vi "RunInference.vi"(4 "Output Index":i32, 6 "Input Index":i32, 7 "DLL path":path, 8 "error in (no error)":errorcluster, 9 "Output Buffer":sgl[](array[numeric]), 10 "Input Buffer":sgl[](array[numeric]), 11 "session id in":i32) -> (0 "error out":errorcluster, 2 "outputBuffer":sgl[](array[numeric]), 3 "session id out":i32)   [LabVIEW 2017, in "ONNX Class Library.lvlib"]
doc: "/**\n * @brief Выполнить инференс (предсказание) модели\n * \n * Основная функция для получения предсказания от модели. Принимает входные данные,\n * передаёт их в нейросеть и записывает результат в выходной буфер.\n * \n * @param sessionId [IN] ID сессии\n * @param inputIndex [IN] Индекс входа (обычно 0 для моделей с одним входом)\n * @param inputBuffer [IN] Массив входных данных (тип должен соответствовать GetInputType)\n * @param inputSize [IN] Количество элементов во входном массиве\n * @param outputIndex [IN] Индекс выхода (обычно 0 для моделей с одним выходом)\n * @param outputBuffer [OUT] Массив для записи результатов (должен быть выделен в LabVIEW)\n * @param outputSize [IN] Размер выходного буфера в элементах\n * \n * @return int32: 0 при успешном выполнении инференса\n * @return int32: -1 при ошибке (сессия не загружена, неверные индексы, ошибка ONNX Runtime)\n * \n * @note Входные данные должны быть нормализованы так же, как при обучении модели\n * @note Размер входного массива должен соответствовать произведению всех размерностей shape\n * @note Выходной буфер должен быть достаточного размера (см. GetOutputShapeDim)\n * @note Функция блокирует выполнение до завершения инференса\n * \n * @example\n * // Для модели с входом [1, 10] и выходом [1, 3]:\n * float inputData[10] = {...};\n * float outputData[3];\n * RunInference(sessionId, 0, inputData, 10, 0, outputData, 3);\n */\nint RunInference(int sessionId, int inputIndex, float* inputBuffer, int inputSize, \n int outputIndex, float* outputBuffer, int outputSize);"
uses:
  ONNX Class Library.lvlib
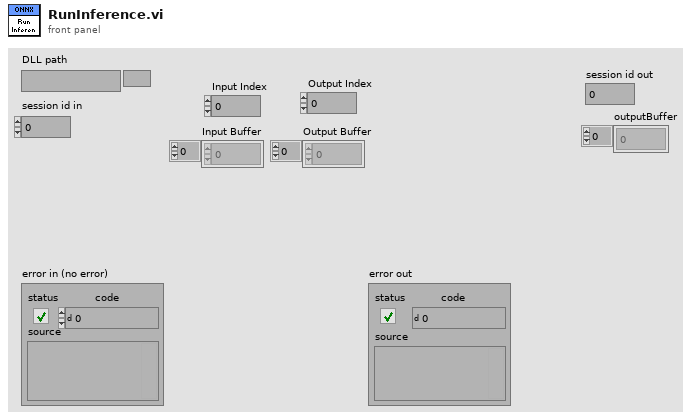
[diagram p1: front panel]
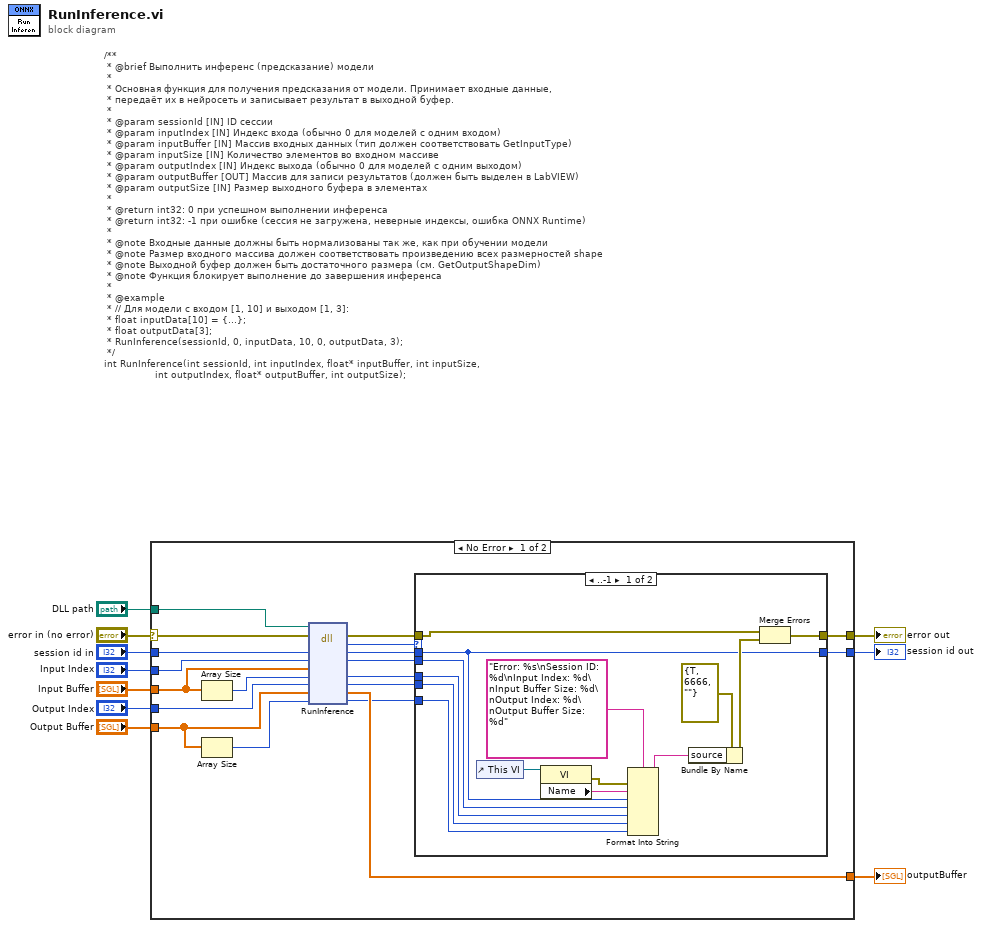
[diagram p0: block diagram]
diagram:
  # "/**\n * @brief Выполнить инференс (предсказание) модели\n * \n * Основная функция для получения предсказания от модели. Принимает входные данные,\n * передаёт их в нейросеть и записывает результат в выходной буфер.\n * \n * @param sessionId [IN] ID сессии\n * @param inputIndex [IN] Индекс входа (обычно 0 для моделей с одним входом)\n * @param inputBuffer [IN] Массив входных данных (тип должен соответствовать GetInputType)\n * @param inputSize [IN] Количество элементов во входном массиве\n * @param outputIndex [IN] Индекс выхода (обычно 0 для моделей с одним выходом)\n * @param outputBuffer [OUT] Массив для записи результатов (должен быть выделен в LabVIEW)\n * @param outputSize [IN] Размер выходного буфера в элементах\n * \n * @return int32: 0 при успешном выполнении инференса\n * @return int32: -1 при ошибке (сессия не загружена, неверные индексы, ошибка ONNX Runtime)\n * \n * @note Входные данные должны быть нормализованы так же, как при обучении модели\n * @note Размер входного массива должен соответствовать произведению всех размерностей shape\n * @note Выходной буфер должен быть достаточного размера (см. GetOutputShapeDim)\n * @note Функция блокирует выполнение до завершения инференса\n * \n * @example\n * // Для модели с входом [1, 10] и выходом [1, 3]:\n * float inputData[10] = {...};\n * float outputData[3];\n * RunInference(sessionId, 0, inputData, 10, 0, outputData, 3);\n */\nint RunInference(int sessionId, int inputIndex, float* inputBuffer, int inputSize, \n                 int outputIndex, float* outputBuffer, int outputSize);"
  n1 = case shown="No Error" "error in (no error)" {
    selector: "error in (no error)" -> [w13 w47]
    tunnel: "session id in" -> [w29 w46]
    tunnel: "Input Index" -> [w28 _]
    tunnel: "Input Buffer" -> [w27 _]
    tunnel: [w25 _] -> w7
    tunnel: "Output Index" -> [w24 _]
    tunnel: [w20 w47] -> w5
    tunnel: [w19 w46] -> w4
    tunnel: "DLL path" -> [w14 _]
    tunnel: "Output Buffer" -> [w12 _]
    frame No Error {
      n2 = Array Size(array=w27) -> (size(s)=w26:i32)
      n3 = Array Size(array=w12) -> (size(s)=w11:i32)
      n4 = dll-call lib="home/ivan/LabVIEWData/ONNX/Test/libonnx_wrapper/unix64/libonnx_wrapper.*" fn="RunInference"(path in=w14, error in=w13, "sessionId"=w29, "inputIndex"=w28, "inputBuffer"=w27, "inputSize"=w26, "outputIndex"=w24, "outputBuffer"=w12, "outputSize"=w11) -> (error out=w23:errorcluster, "return"=w22:i32, "sessionId"=w21:i32, "inputIndex"=w18:i32, "inputSize"=w17:i32, "outputIndex"=w16:i32, "outputBuffer"=w25:sgl[], "outputSize"=w15:i32)  [unwired: 2 in, 1 out]
      n5 = case shown="..-1" w22 {
        tunnel: w23 -> [w34 w45]
        tunnel: [w35 w45] -> w20
        tunnel: w21 -> [w36 w44]
        tunnel: [w36 w44] -> w19
        tunnel: w18 -> [w33 _]
        tunnel: w17 -> [w32 _]
        tunnel: w16 -> [w31 _]
        tunnel: w15 -> [w30 _]
        frame ..-1 {
          n6 = control-ref of="This VI"() -> (w40:refnum<vi>)
          n7 = property class="VI"(reference=w40) -> (error out=w37:errorcluster, "Name"=w39:string)  [unwired: 1 in, 1 out]
          n8 = Format Into String(format string="Error: %s\nSession ID: %d\nInput Index: %d\nInput Buffer Size: %d\nOutput Index: %d\nOutput Buffer Size: %d", error in=w37, w39, w36, w33, w32, w31, w30) -> (resulting string=w41:string)  [unwired: 1 in, 1 out]
          n9 = Bundle By Name(cluster=errorcluster {"status"=TRUE, "code"=6666, "source"=""} ("error out"), "source"=w41) -> (w42:errorcluster)
          n10 = Merge Errors(w34, w42) -> (w35:errorcluster)
        }
        frame 0.. {
        }
      }
    }
    frame Error {
    }
  }
  "error out" <- w5
  "session id out" <- w4
  "outputBuffer" <- w7
